vi "set_FPGA_reference.vi"(8 "error in (no error)":errorcluster, 10 "FPGA interface":refnum<k20>, 11 "GenericFPGAWrapper in":refnum<class "GenericFPGAWrapper.lvclass">) -> (0 "error out":errorcluster, 3 "GenericFPGAWrapper out":refnum<class "GenericFPGAWrapper.lvclass">)   [LabVIEW 2010]
uses:
  GenericFPGAWrapper.lvclass
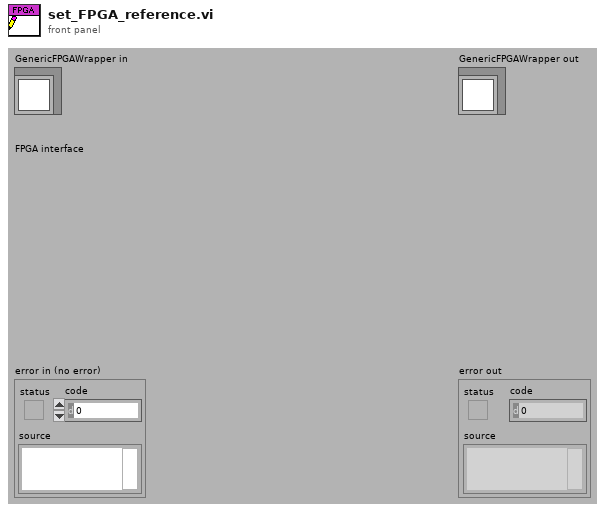
[diagram p1: front panel]
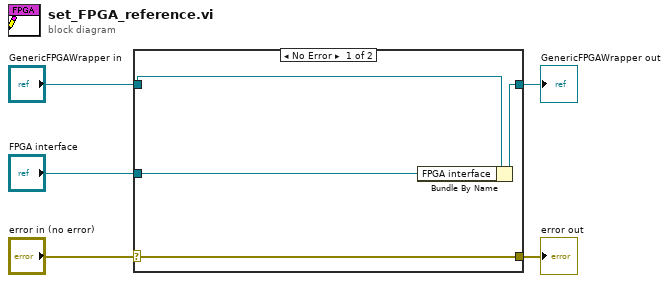
[diagram p0: block diagram]
diagram:
  n1 = case shown="No Error" "error in (no error)" {
    selector: "error in (no error)" -> [w9 w10]
    tunnel: [w9 w10] -> w4
    tunnel: [w7 w11] -> w2
    tunnel: "GenericFPGAWrapper in" -> [w8 w11]
    tunnel: "FPGA interface" -> [w6 _]
    frame No Error {
      n2 = Bundle By Name(cluster=w8, "FPGA interface"=w6) -> (w7:refnum<class "GenericFPGAWrapper.lvclass">)
    }
    frame Error {
    }
  }
  "error out" <- w4
  "GenericFPGAWrapper out" <- w2
